vi "programa 8.vi"() -> ()   [LabVIEW 2011]
panel:
  out "Contador":dbl
  out "Temp 36-60":dbl
  out "Temp 21-35":dbl
  out "Temp 1-20":dbl
  out "Temperatura":i32(slide) scale=0.0..60.0
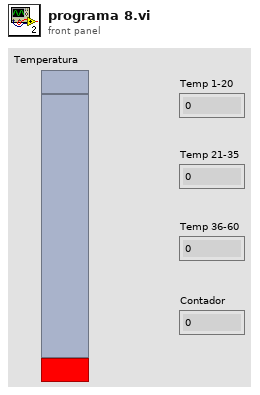
[diagram p1: front panel]
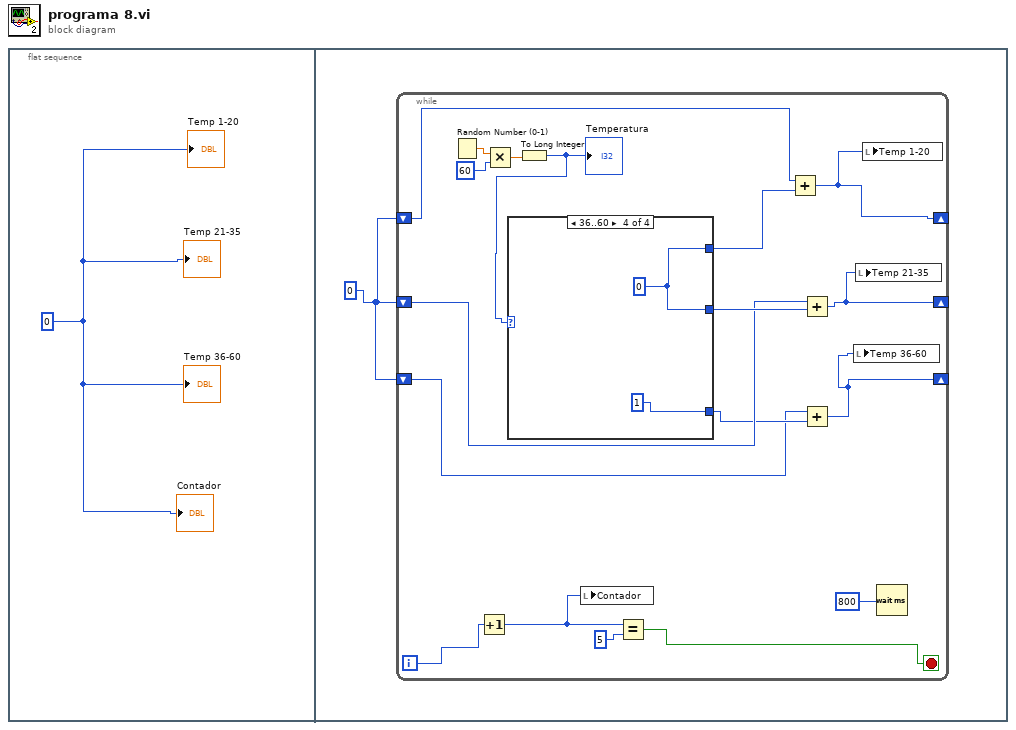
[diagram p0: block diagram]
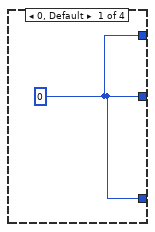
[diagram p2: hidden frame]
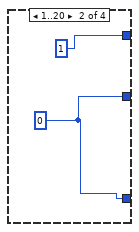
[diagram p3: hidden frame]
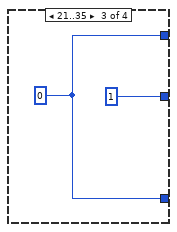
[diagram p4: hidden frame]
diagram:
  n1 = flat-sequence {
    frame #0 {
      w1 = 0
      "Contador" <- w1
      "Temp 1-20" <- w1
      "Temp 21-35" <- w1
      "Temp 36-60" <- w1
    }
    frame #1 {
      w2 = 0
      n2 = while {
        shift-right: [w4] -> _
        shift-left: w2 -> [w11]
        shift-right: [w5] -> _
        shift-left: w2 -> [w8]
        shift-right: [w3] -> _
        shift-left: w2 -> [w6]
        i -> [w20]
        stop <- w14 stop-if-true
        n3 = Random Number (0-1)() -> (number: 0 to 1=w18:dbl)
        n4 = Increment(x=w20) -> (x+1=w15:i32)
        n5 = Multiply(x=w18, y=60) -> (x*y=w17:dbl)
        n6 = To Long Integer(number=w17) -> (32bit integer=w13:i32)
        "Temperatura" <- w13
        n7 = case shown="36..60" w13 {
          tunnel: [w21 w22 1 w26] -> w10
          tunnel: [w21 1 w24 w26] -> w9
          tunnel: [w21 w22 w24 1] -> w7
          frame 0, Default {
            w21 = 0
          }
          frame 1..20 {
            w22 = 0
          }
          frame 21..35 {
            w24 = 0
          }
          frame 36..60 {
            w26 = 0
          }
        }
        n8 = local write "Contador"(w15) -> ()
        n9 = Equal?(x=w15, y=5) -> (x = y?=w14:bool)
        n10 = Add(x=w11, y=w9) -> (x+y=w4:i32)
        n11 = Add(x=w8, y=w10) -> (x+y=w5:i32)
        n12 = Add(x=w6, y=w7) -> (x+y=w3:i32)
        n13 = local write "Temp 36-60"(w3) -> ()
        n14 = local write "Temp 21-35"(w5) -> ()
        n15 = local write "Temp 1-20"(w4) -> ()
        n16 = Wait (ms)(milliseconds to wait=800) -> ()  [unwired: 1 out]
      }
    }
  }
